vi "GTCP331-200ER - 1.C.(9).vi"(8 "error in (no error)":errorcluster, 11 "RT - Analysis Data in in in":T1={"Accel Sensistivity"=[0.0, 0.0, 0.0], "Cutoff Frequncies"=[{"LP Passband"=0.0, "HP Stopband"=0.0, "LP Stopband"=0.0, "HP Passband"=0.0}, {"LP Passband"=0.0, "HP Stopband"=0.0, "LP Stopband"=0.0, "HP Passband"=0.0}, {"LP Passband"=0.0, "HP Stopband"=0.0, "LP Stopband"=0.0, "HP Passband"=0.0}], "APU Setup File"={"Sensor Info"=[], "Calibration Info"=[], "CMM Table 106"=[], "CMM Table 106B "=[], "Accel Config"=[], "Report Sheet 1"=[], "Report Sheet 2"=[], "Report Sheet 3"=[]}, "RepairLevel"=""} {"Cutoff Frequncies"."HP Passband" min=1.0 step=1.0 format="%#.4f"; "Cutoff Frequncies"."LP Stopband" min=1.0 step=1.0 format="%#.4f"; "Cutoff Frequncies"."HP Stopband" min=1.0 step=1.0 format="%#.4f"; "Cutoff Frequncies"."LP Passband" min=1.0 step=1.0 format="%#.4f"}) -> (0 "error out":errorcluster, 2 "Interactive Mode Vals":dbl[](array[numeric]), 3 "RT - Analysis Data in out":T1 {"Cutoff Frequncies"."HP Passband" min=1.0 step=1.0 format="%#.4f"; "Cutoff Frequncies"."LP Stopband" min=1.0 step=1.0 format="%#.4f"; "Cutoff Frequncies"."HP Stopband" min=1.0 step=1.0 format="%#.4f"; "Cutoff Frequncies"."LP Passband" min=1.0 step=1.0 format="%#.4f"})   [LabVIEW 2018, in "RT - Analysis.lvlib"]
doc: "This subtest perfmors engine run-in procedures."
uses:
  RT - Analysis.lvlib
  Private Controls/Watchdog Settings.ctl
  Private Controls/RT-Analysis Data.ctl
  Modules/Testing UI 3/Private Controls/Cutoff Frequency.ctl
  Modules/Testing UI 3/Testing UI 3.lvlib
  Top Level/Shared Controls/APU Setup File.ctl
panel:
  # "Highpass Cutoff Frequency"
  # "Lowpass Cutoff Frequency"
  # "Highpass Cutoff Frequency"
  # "Lowpass Cutoff Frequency"
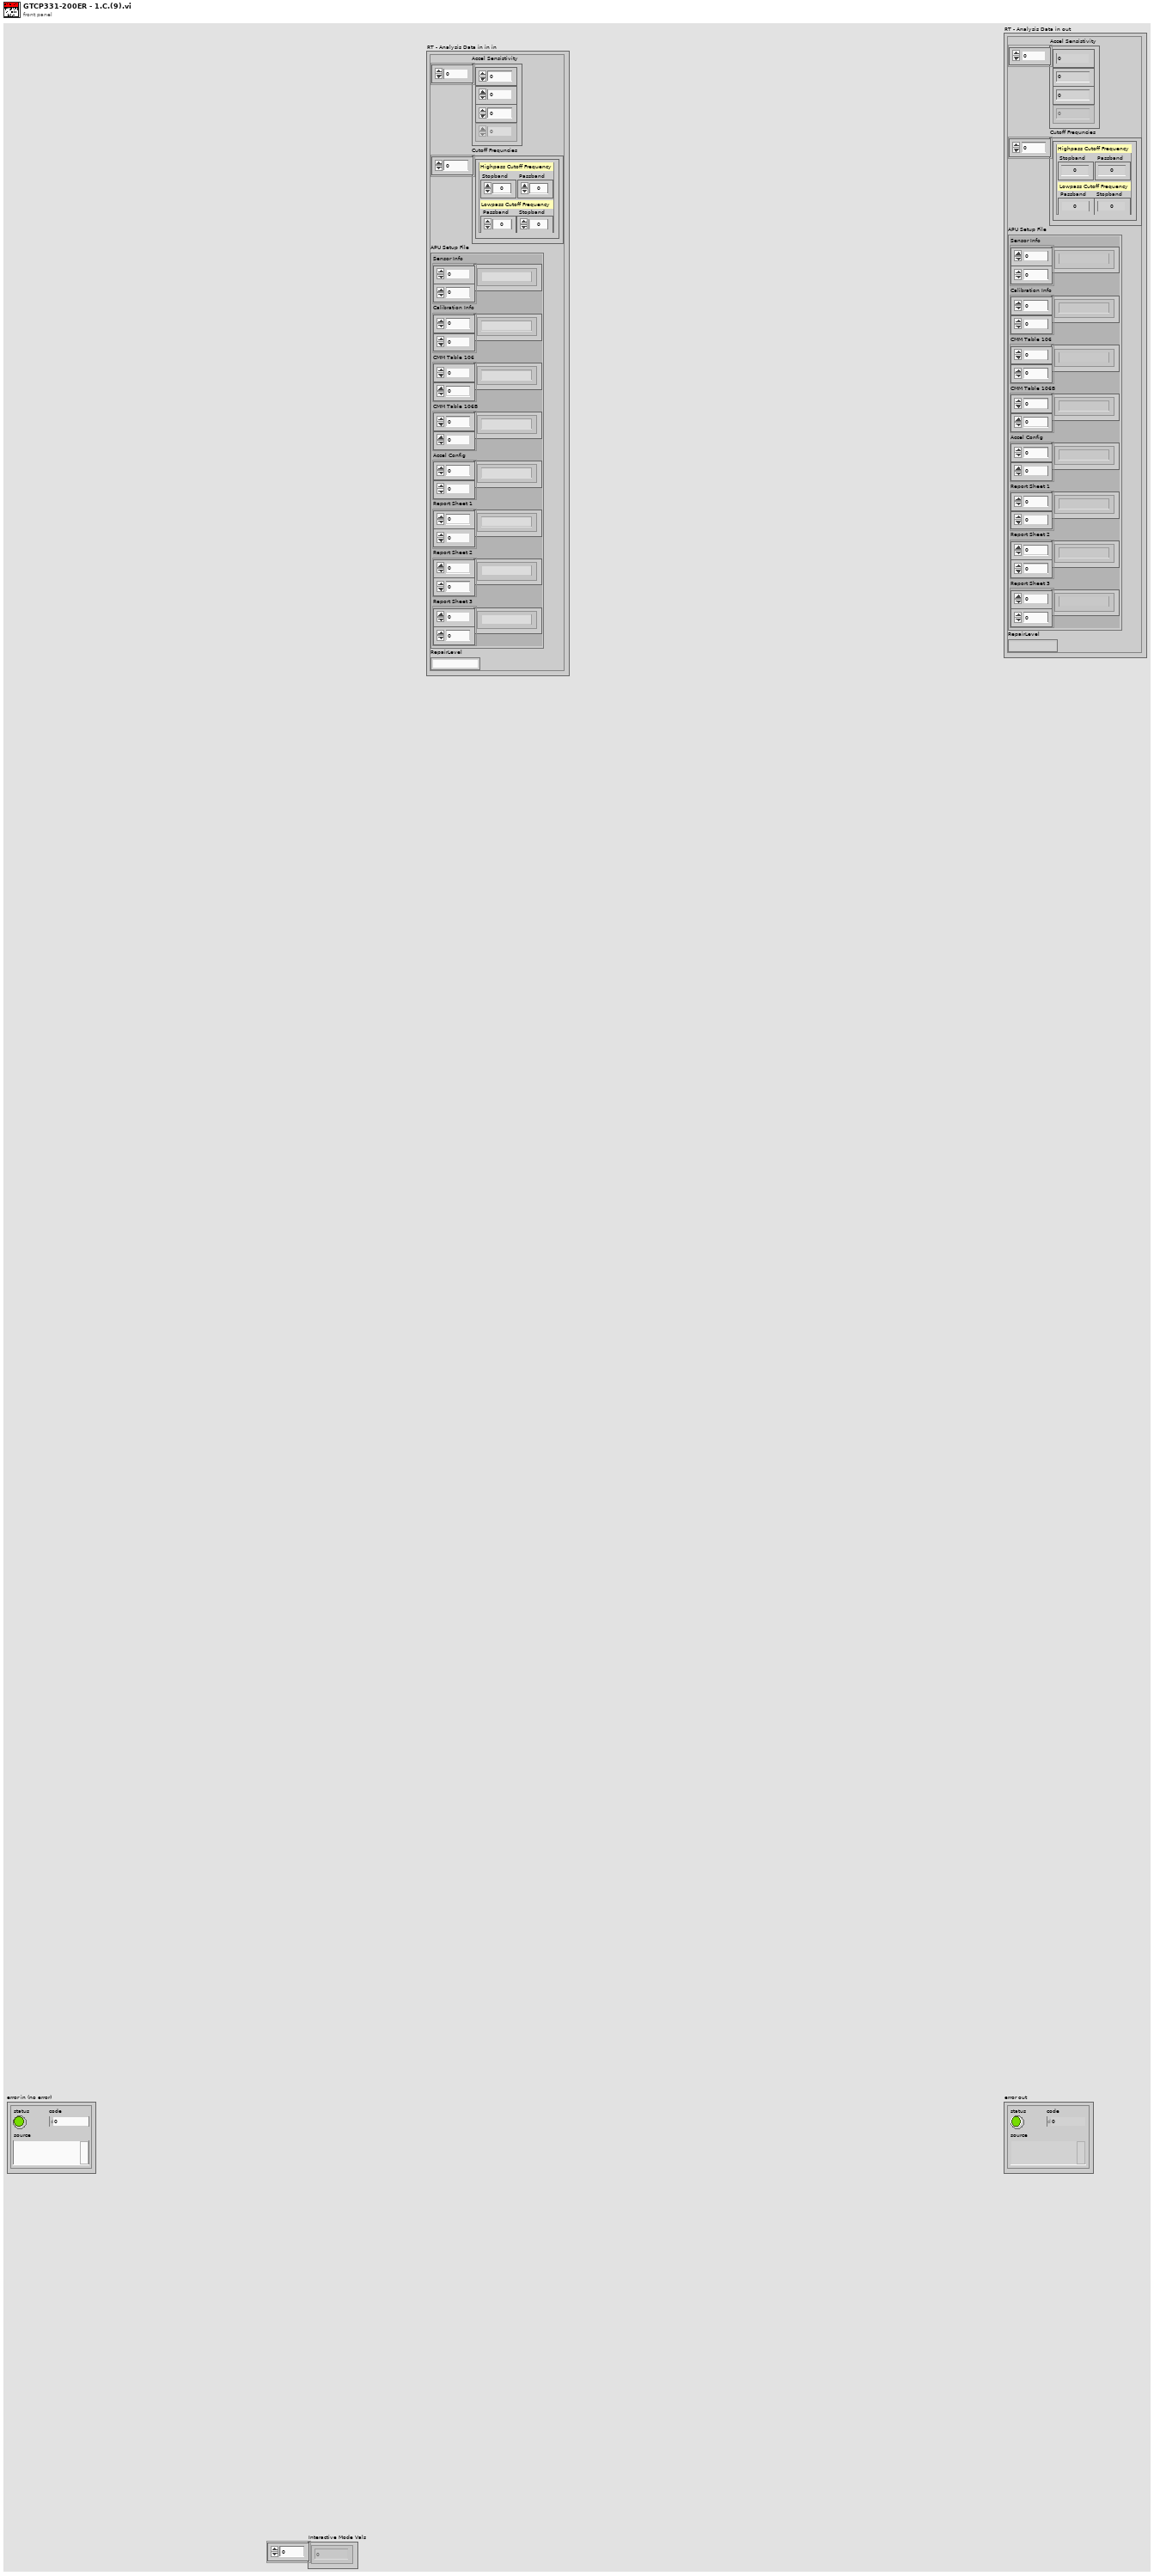
[diagram p1: front panel]
types:
  T1 = typedef "RT - Analysis.lvlib/RT-Analysis Data.ctl" = cluster{"Accel Sensistivity":dbl[], "Cutoff Frequncies":T2[], "APU Setup File":T3, "RepairLevel":string}
  T2 = typedef "Testing UI 3.lvlib/Cutoff Frequency.ctl" = cluster{"LP Passband":dbl, "HP Stopband":dbl, "LP Stopband":dbl, "HP Passband":dbl}
  T3 = typedef "APU Setup File.ctl" = cluster{"Sensor Info":string[][], "Calibration Info":string[][], "CMM Table 106":string[][], "CMM Table 106B ":string[][], "Accel Config":string[][], "Report Sheet 1":string[][], "Report Sheet 2":string[][], "Report Sheet 3":string[][]}
  T4 = typedef "RT - Analysis.lvlib/Watchdog Settings.ctl" = cluster{"Watchdog Action":enum16{"Disabled", "Timer - Change Sample Rate", "RPM Thresh - Insert Other", "RPM Thresh - Check POPD", "RPM Thresh - StartStop Logging"}, "Timer Start":timestamp, "[Watchdog Bools]":bool[], "[Watchdog DBLs]":dbl[], "Watchdog Variant":variant}
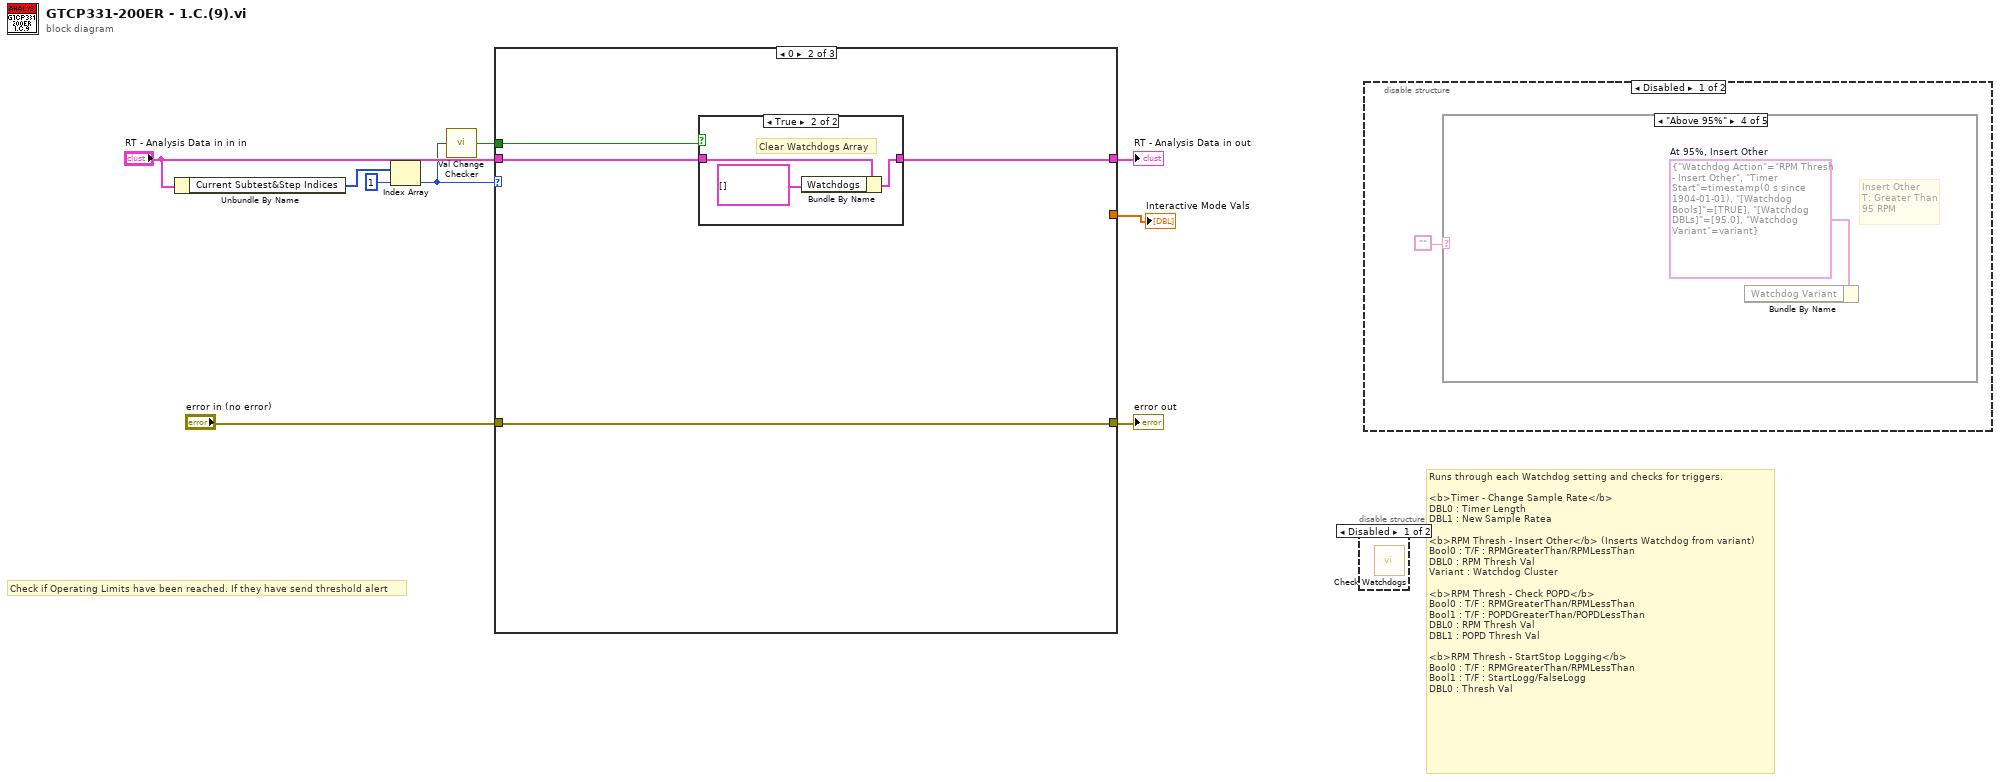
[diagram p0: block diagram]
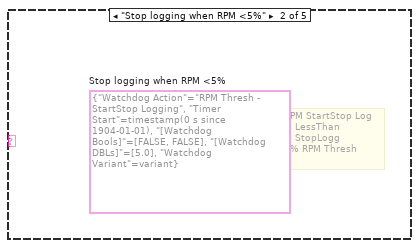
[diagram p3: hidden frame]
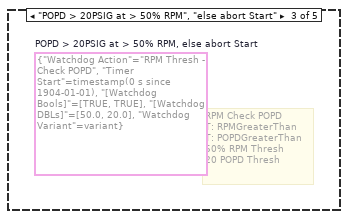
[diagram p4: hidden frame]
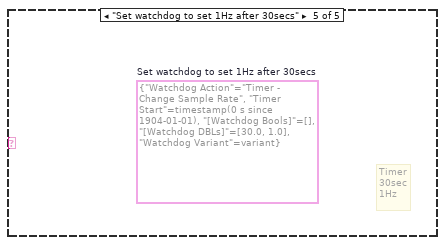
[diagram p5: hidden frame]
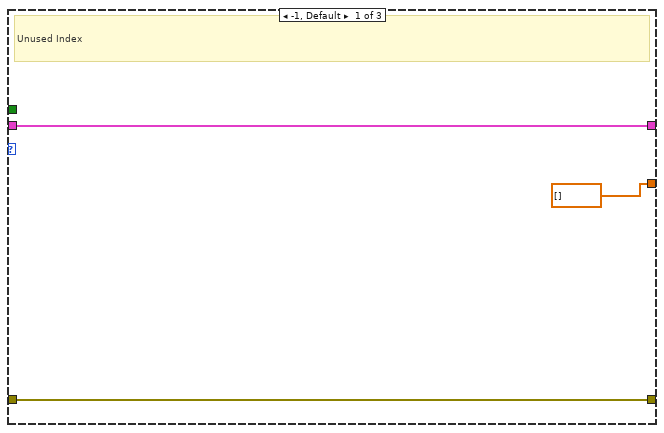
[diagram p8: hidden frame]
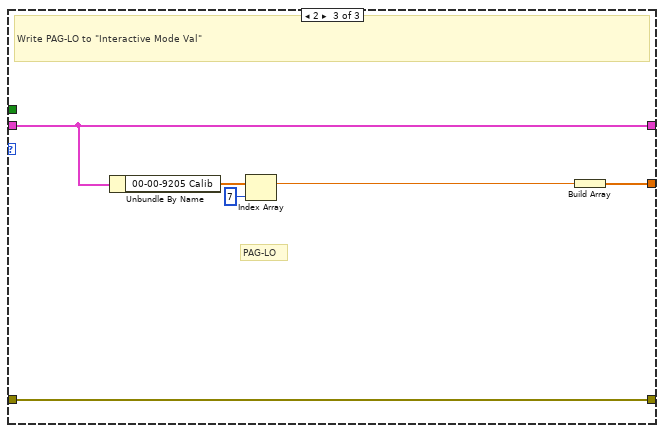
[diagram p10: hidden frame]
diagram:
  # "Runs through each Watchdog setting and checks for triggers.\n\n<b>Timer - Change Sample Rate</b>\nDBL0 : Timer Length\nDBL1 : New Sample Ratea\n\n<b>RPM Thresh - Insert Other</b> (Inserts Watchdog from variant)\nBool0 : T/F : RPMGreaterThan/RPMLessThan\nDBL0 : RPM Thresh Val\nVariant : Watchdog Cluster\n\n<b>RPM Thresh - Check POPD</b>\nBool0 : T/F : RPMGreaterThan/RPMLessThan\nBool1 : T/F : POPDGreaterThan/POPDLessThan\nDBL0 : RPM Thresh Val\nDBL1 : POPD Thresh Val\n\n<b>RPM Thresh - StartStop Logging</b>\nBool0 : T/F : RPMGreaterThan/RPMLessThan\nBool1 : T/F : StartLogg/FalseLogg\nDBL0 : Thresh Val"
  # "Check if Operating Limits have been reached. If they have send threshold alert"
  n1 = Unbundle By Name("RT - Analysis Data in in in") -> ("Current Subtest&Step Indices"=w9:i32[])
  n2 = Index Array(array=w9, index=1) -> (element=w4:i32)
  n3 = call "Val Change Checker.vi"("Current Value in"=w4) -> ("Value Change?"=w3:bool)
  n4 = case shown="0" w4 {
    tunnel: [w12 w16 w26] -> w7
    tunnel: "error in (no error)" -> [w12 w16 w26]
    tunnel: [w11 w14 w25] -> w6
    tunnel: "RT - Analysis Data in in in" -> [w11 w15 w25]
    tunnel: [dbl[] [] ("Interactive Mode Vals") _ w23] -> w1
    tunnel: w3 -> [_ w13 _]
    frame -1, Default {
      # "Unused Index"
    }
    frame 0 {
      n5 = case shown="True" w13 {
        tunnel: w15 -> [w17 w20]
        tunnel: [w17 w19] -> w14
        frame False {
        }
        frame True {
          # "Clear Watchdogs Array"
          n6 = Bundle By Name(cluster=w20, "Watchdogs"=T4[] []) -> (w19:T1)
        }
      }
    }
    frame 2 {
      # "PAG-LO"
      # "Write PAG-LO to \"Interactive Mode Val\""
      n7 = Unbundle By Name(w25) -> ("00-00-9205 Calib"=w24:dbl[])
      n8 = Index Array(array=w24, index=7) -> (element=w22:dbl)
      n9 = Build Array(w22) -> (w23:dbl[])
    }
  }
  "RT - Analysis Data in out" <- w6
  "error out" <- w7
  "Interactive Mode Vals" <- w1
  n10 = disable-structure shown="Disabled" {
    frame Disabled {
      n11 = call "Check Watchdogs.vi"() -> ()  [unwired: 10 in, 2 out]
    }
    frame Enabled {
    }
  }
  n12 = disable-structure shown="Disabled" {
    frame Disabled {
      n13 = case shown="\"Above 95%\"" "" {
        frame Default {
        }
        frame "Stop logging when RPM <5%" {
          (unwired) T4 {"Watchdog Action"=enum."RPM Thresh - StartStop Logging", "Timer Start"=timestamp(0 s since 1904-01-01), "[Watchdog Bools]"=[FALSE, FALSE], "[Watchdog DBLs]"=[5.0], "Watchdog Variant"=variant}  # Stop logging when RPM <5%
          # "RPM StartStop Log\nF: LessThan\nF: StopLogg\n5% RPM Thresh"
        }
        frame "POPD > 20PSIG at > 50% RPM", "else abort Start" {
          (unwired) T4 {"Watchdog Action"=enum."RPM Thresh - Check POPD", "Timer Start"=timestamp(0 s since 1904-01-01), "[Watchdog Bools]"=[TRUE, TRUE], "[Watchdog DBLs]"=[50.0, 20.0], "Watchdog Variant"=variant}  # POPD > 20PSIG at > 50% RPM, else abort Start
          # "RPM Check POPD\nT: RPMGreaterThan\nT: POPDGreaterThan\n50% RPM Thresh\n20 POPD Thresh"
        }
        frame "Above 95%" {
          w28 = T4 {"Watchdog Action"=enum."RPM Thresh - Insert Other", "Timer Start"=timestamp(0 s since 1904-01-01), "[Watchdog Bools]"=[TRUE], "[Watchdog DBLs]"=[95.0], "Watchdog Variant"=variant}  # At 95%, Insert Other
          # "Insert Other\nT: Greater Than\n95 RPM"
          n14 = Bundle By Name(cluster=w28) -> ()  [unwired: 1 in, 1 out]
        }
        frame "Set watchdog to set 1Hz after 30secs" {
          (unwired) T4 {"Watchdog Action"=enum."Timer - Change Sample Rate", "Timer Start"=timestamp(0 s since 1904-01-01), "[Watchdog Bools]"=[], "[Watchdog DBLs]"=[30.0, 1.0], "Watchdog Variant"=variant}  # Set watchdog to set 1Hz after 30secs
          # "Timer\n30sec\n1Hz"
        }
      }
    }
    frame Enabled {
    }
  }
